vi "finde alle.vi"(0 "Array":dbl[](array[numeric]), 7 "element":dbl) -> (4 "Indizes":i32[](array[numeric]))   [LabVIEW 2010, in "util.lvlib"]
uses:
  util.lvlib
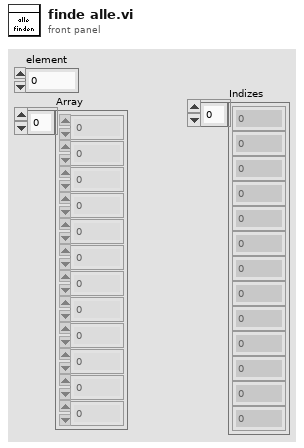
[diagram p1: front panel]
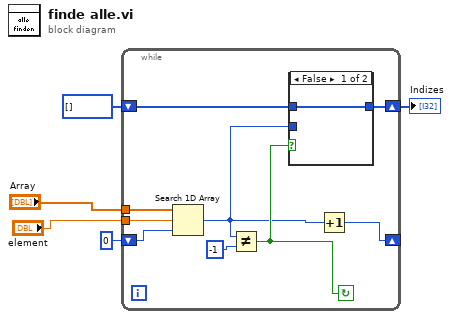
[diagram p0: block diagram]
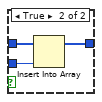
[diagram p2: hidden frame]
diagram:
  n1 = while {
    tunnel: "Array" -> [w14]
    shift-right: [w6] -> _
    shift-left: 0 ("index of element") -> [w12]
    tunnel: "element" -> [w11]
    shift-right: [w9] -> w1
    shift-left: i32[] [] -> [w8]
    stop <- w10 continue-if-true
    n2 = Search 1D Array(1D array=w14, element=w11, start index (0)=w12) -> (index of element=w7:i32)
    n3 = Not Equal?(x=w7, y=-1) -> (x != y?=w10:bool)
    n4 = case shown="False" w10 {
      tunnel: w7 -> [_ w18]
      tunnel: [w15 w17] -> w9
      tunnel: w8 -> [w15 w16]
      frame False {
      }
      frame True {
        n5 = Insert Into Array(array=w16, new element=w18) -> (w17:i32[])  [unwired: 1 in]
      }
    }
    n6 = Increment(x=w7) -> (x+1=w6:i32)
  }
  "Indizes" <- w1
